vi "Make Hardware Connect Calls.vi"(8 "error in (no error)":errorcluster, 11 "Engine Run Time Data in":T1) -> (0 "error out":errorcluster, 3 "Engine Run Time Data out":T1)   [LabVIEW 2023, in "NI 272x Resistive Simulation Custom Device Engine.lvlib"]
uses:
  NI 272x Resistive Simulation Custom Device Engine.lvlib
  <instrlib>/ni272xReferenceVIs/ni272xReferenceVIs.llb/ni272x Disconnect 2Chan.vi
  <instrlib>/ni272xReferenceVIs/ni272xReferenceVIs.llb/ni272x Connect 2Chan.vi
  Controls/Channel Mode.ctl
  NI 272x Resistive Simulation Custom Device Shared.lvlib
  <instrlib>/ni272xReferenceVIs/ni272xReferenceVIs.llb/ni272x Callendar-Van Dusen RTD Parameters.ctl
  Controls/Compiled HW Channel.ctl
  Controls/Compiled Connect Channel.ctl
  Controls/Compiled Engine Data.ctl
  <instrlib>/ni272xReferenceVIs/ni272xReferenceVIs.llb/ni272x Reference.ctl
  Controls/Engine Run Time Data.ctl
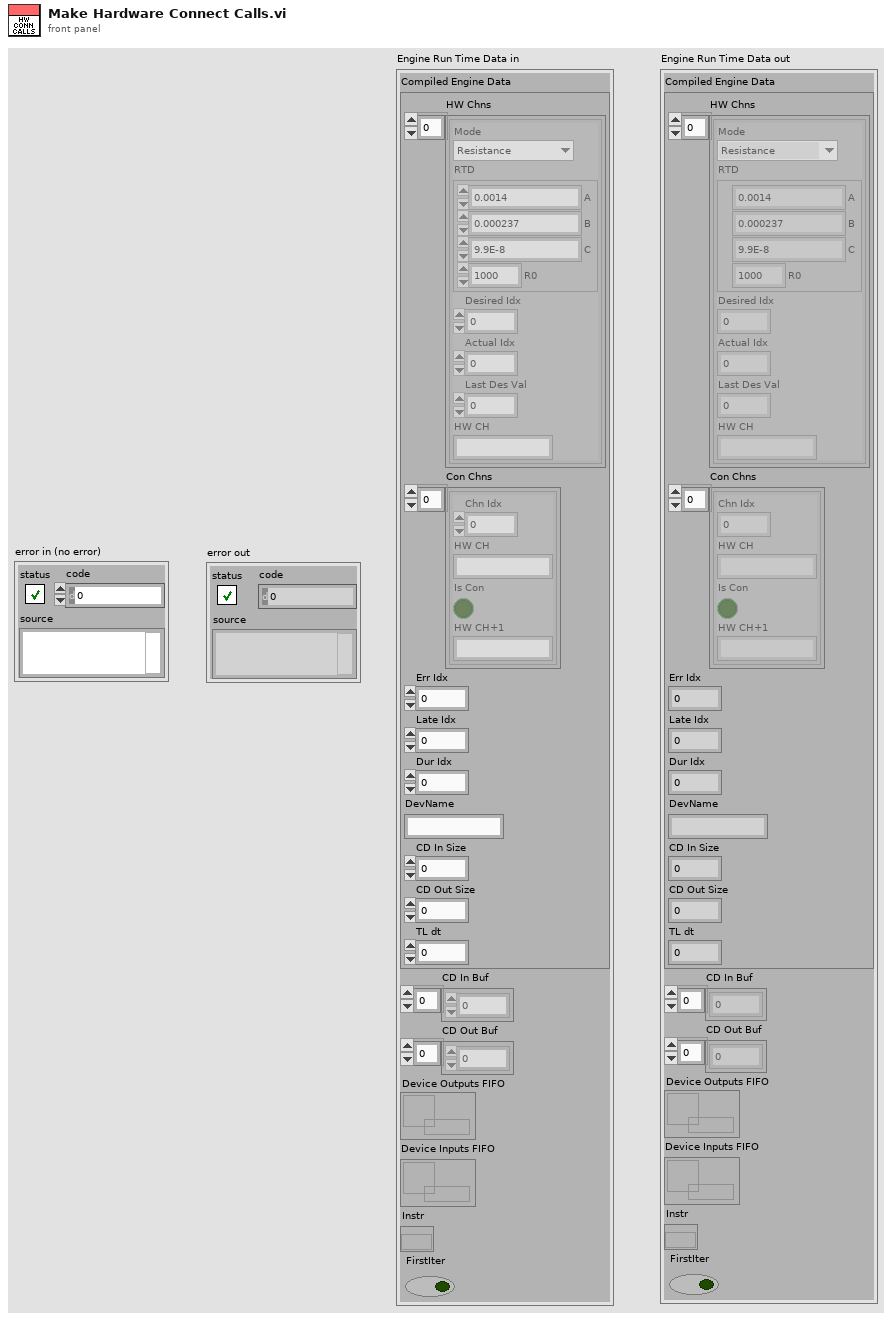
[diagram p1: front panel]
types:
  T1 = typedef "NI 272x Resistive Simulation Custom Device Engine.lvlib/Engine Run Time Data.ctl" = cluster{"Compiled Engine Data":T2, "CD In Buf":dbl[], "CD Out Buf":dbl[], "Device Outputs FIFO":refnum<k33>, "Device Inputs FIFO":refnum<k33>, "Instr":T7, "FirstIter":bool}
  T2 = typedef "NI 272x Resistive Simulation Custom Device Shared.lvlib/Compiled Engine Data.ctl" = cluster{"HW Chns":T3[], "Con Chns":T6[], "Err Idx":i32, "Late Idx":i32, "Dur Idx":i32, "DevName":string, "CD In Size":i32, "CD Out Size":i32, "TL dt":i64}
  T3 = typedef "NI 272x Resistive Simulation Custom Device Shared.lvlib/Compiled HW Channel.ctl" = cluster{"Mode":T4, "RTD":T5, "Desired Idx":i32, "Actual Idx":i32, "Last Des Val":dbl, "HW CH":string}
  T4 = typedef "NI 272x Resistive Simulation Custom Device Shared.lvlib/Channel Mode.ctl" = enum16{"Resistance", "RTD Temperature"}
  T5 = typedef "ni272x Callendar-Van Dusen RTD Parameters.ctl" = cluster{"A":dbl, "B":dbl, "C":dbl, "R0":dbl}
  T6 = typedef "NI 272x Resistive Simulation Custom Device Shared.lvlib/Compiled Connect Channel.ctl" = cluster{"Chn Idx":i32, "HW CH":string, "Is Con":bool, "HW CH+1":string}
  T7 = typedef "ni272x Reference.ctl" = refnum<k20>
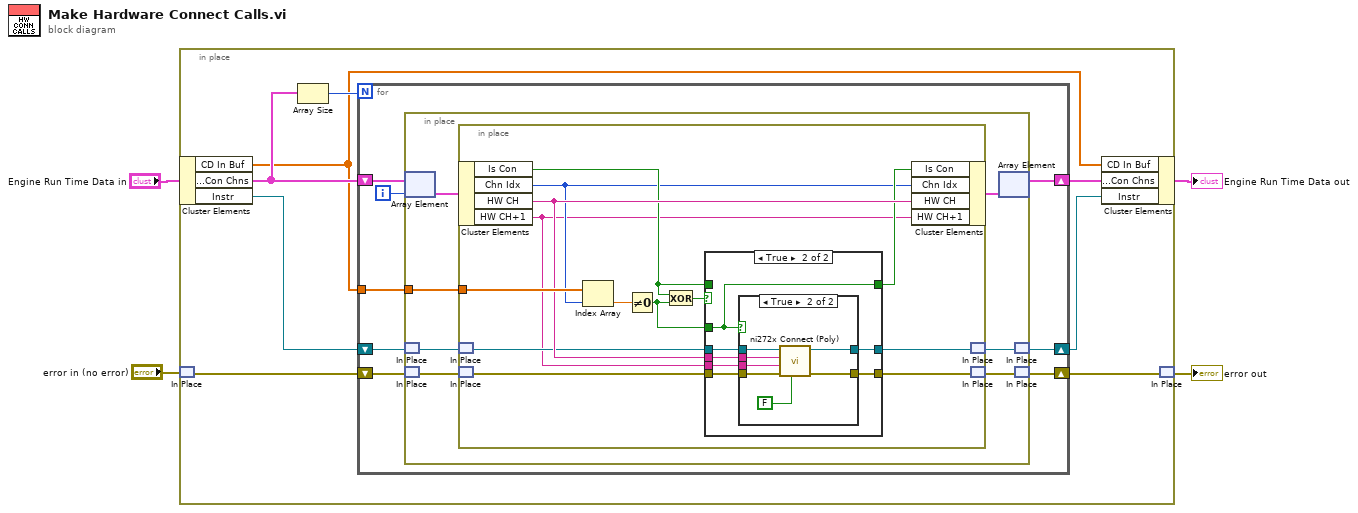
[diagram p0: block diagram]
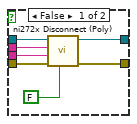
[diagram p3: hidden frame]
diagram:
  n1 = in-place {
    n2 = in-place-cluster #1("Engine Run Time Data in") -> ("CD In Buf"=w8:dbl[], "Compiled Engine Data.Con Chns"=w9:T6[], "Instr"=w12:T7)
    n3 = in-place-match #2("error in (no error)") -> (w11:errorcluster)
    n4 = Array Size(array=w9) -> (size(s)=w10:i32)
    n5 = for {
      N: w10 -> [_]
      tunnel: w8 -> [w18]
      shift-right: [w14] -> w6
      shift-left: w12 -> [w15]
      shift-right: [w16] -> w5
      shift-left: w11 -> [w17]
      shift-right: [w13] -> w7
      shift-left: w9 -> [w20]
      i -> [w19]
      n6 = in-place {
        in-place-border: w18 -> [w26]
        n7 = in-place-array #3(w20, w19) -> (w27:T6)
        n8 = in-place-match #4(w15) -> (w22:T7)
        n9 = in-place-match #5(w17) -> (w25:errorcluster)
        n10 = in-place {
          in-place-border: w26 -> [w40]
          n11 = in-place-cluster #6(w27) -> ("Is Con"=w30:bool, "Chn Idx"=w29:i32, "HW CH"=w39:string, "HW CH+1"=w28:string)
          n12 = in-place-match #7(w22) -> (w36:T7)
          n13 = in-place-match #8(w25) -> (w38:errorcluster)
          n14 = Index Array(array=w40, index=w29) -> (element=w34:dbl)
          n15 = Not Equal To 0?(x=w34) -> (x != 0?=w32:bool)
          n16 = Exclusive Or(1:w32, 2:w30) -> (0:w33:bool)
          n17 = case shown="True" w33 {
            tunnel: w39 -> [_ w48]
            tunnel: w38 -> [w43 w50]
            tunnel: w36 -> [w42 w49]
            tunnel: [w43 w47] -> w37
            tunnel: [w42 w46] -> w35
            tunnel: w28 -> [_ w45]
            tunnel: w32 -> [_ w44]
            tunnel: [w41 w44] -> w31
            tunnel: w30 -> [w41 _]
            frame False {
            }
            frame True {
              n18 = case shown="True" w44 {
                tunnel: w50 -> [w57 w64]
                tunnel: w49 -> [w56 w61]
                tunnel: w48 -> [w55 w60]
                tunnel: [w51 w63] -> w47
                tunnel: [w52 w62] -> w46
                tunnel: w45 -> [w54 w59]
                frame False {
                  n19 = call-poly <instrlib>:"ni272x Disconnect (Poly).vi"("wait for settling (T)"=FALSE, "error in (no error)"=w57, "resistor channel N+1"=w54, "resistor channel N"=w55, "instrument handle"=w56) -> ("error out"=w51:errorcluster, "instrument handle out"=w52:T7)  [unwired: 5 out]
                }
                frame True {
                  n20 = call-poly <instrlib>:"ni272x Connect (Poly).vi"("wait for settling (T)"=FALSE, "error in (no error)"=w64, "resistor channel N+1"=w59, "resistor channel N"=w60, "instrument handle"=w61) -> ("error out"=w63:errorcluster, "instrument handle out"=w62:T7)  [unwired: 5 out]
                }
              }
            }
          }
          n21 = in-place-cluster #6("Is Con"=w31, "Chn Idx"=w29, "HW CH"=w39, "HW CH+1"=w28) -> (w23:T6)
          n22 = in-place-match #7(w35) -> (w21:T7)
          n23 = in-place-match #8(w37) -> (w24:errorcluster)
        }
        n24 = in-place-array #3(w23) -> (w13:T6[])  [unwired: 1 out]
        n25 = in-place-match #4(w21) -> (w14:T7)
        n26 = in-place-match #5(w24) -> (w16:errorcluster)
      }
    }
    n27 = in-place-cluster #1("CD In Buf"=w8, "Compiled Engine Data.Con Chns"=w7, "Instr"=w6) -> (→"Engine Run Time Data out":T1)
    n28 = in-place-match #2(w5) -> (→"error out":errorcluster)
  }
